vi "fgv_AOL_Globals Read.vi"(8 "error in (no error)":errorcluster) -> (0 "error out":errorcluster, 2 "AOL_Globals":T1={"Imaging Protocol"=enum."AOL Z-Stack", "Number of POI"=0, "Number of Miniscans"=0, "Number of Trials"=0, "Number of Cycles "=0, "# Averaged Frames"=0, "Laser power (%)"=0, "Pockels (V)"=0.0, "Acquisition Length (sec)"=0.0, "Fill time (us)"=0.0, "POI Dwell time (us)"=0.0, "Miniscan Dwell time per pixel (us)"=0.0, "PMT 1"=0.0, "PMT 2"=0.0, "Back Apperture (mA)"=0.0, "Frame Size"=512, "Center Frequency"=0.0, "Field of View (um)"=175.0, "Field of View (norm)"=175.0, "DwellTime (us)"=0.0, "Ref Dwell Time (us)"=0.0, "Wavelength (nm)"=0.0, "Zoom"=1.0, "AOL Z"=0.0, "AOL Mode"=enum."Raster", "GridXY"=0.0, "GridZ"=0.0, "TriggerPeriod (sec)"=0.0, "Number of Pixels in Miniscan"=0, "Experiment folder path"=path "", "X centre"=0.0, "Y centre"=0.0, "Angle (degrees)"=0.0, "Angle Xs (degrees)"=0.0, "Angle Ys (degrees)"=0.0, "Plane Mode"=0, "Threshold"=[], "Regenerate Chirps"=FALSE, "Rectangle ROI length (pixels)"=0, "Rectangle ROI height (pixels)"=0, "AOD fill"=4900, "StartupDelay"=0, "Samples Wait after Trigger"=5080, "Slip Cycle"=600000, "Add Cycle"=TRUE, "Functional Mode"=enum."Point", "Z Start"=0.0, "Z Stop"=0.0, "# Planes"=0, "Total Pixels"=0, "Variable Miniscan Pixels"=[], "Use Variable Length"=FALSE, "Use Variable Resolution"=FALSE, "Laser power (%) at Z Start"=0, "Laser power (%) at Z Stop"=0, "Ref Z Step"=0} {"Angle Ys (degrees)" format="%#.6g"; "Angle Xs (degrees)" format="%#.6g"; "Plane Mode" items=["XY Plane", "XZ Plane", "YZ Plane", "arbitraryplane"]; "Frame Size" items=["100X100"=100, "128X128"=128, "200X200"=200, "256X256"=256, "512X512"=512, "1024x1024"=1024, "2048x2048"=2048]; "Back Apperture (mA)" format="%#.6g"; "Pockels (V)" format="%#.6g"; "PMT 2" format="%#.6g"; "PMT 1" format="%#.6g"; "Angle (degrees)" format="%#.6g"; "POI Dwell time (us)" format="%#.6g"}, 3 "Imaging Protocol":T2)   [LabVIEW 2020]
uses:
  Typedefs/Controls/AOL_Globals.ctl
  Typedefs/Imaging Protocols enum.ctl
  Typedefs/Frame Size.ctl
  Typedefs/AOL modes.ctl
  Typedefs/Plane Mode.ctl
  Typedefs/Functional Mode.ctl
panel:
  # "<---- NOTE!  I don't think the PMT1\n          and PMT2 values are used. Elliminate."
  # "<---- NOTE!  Normalised FOV value"
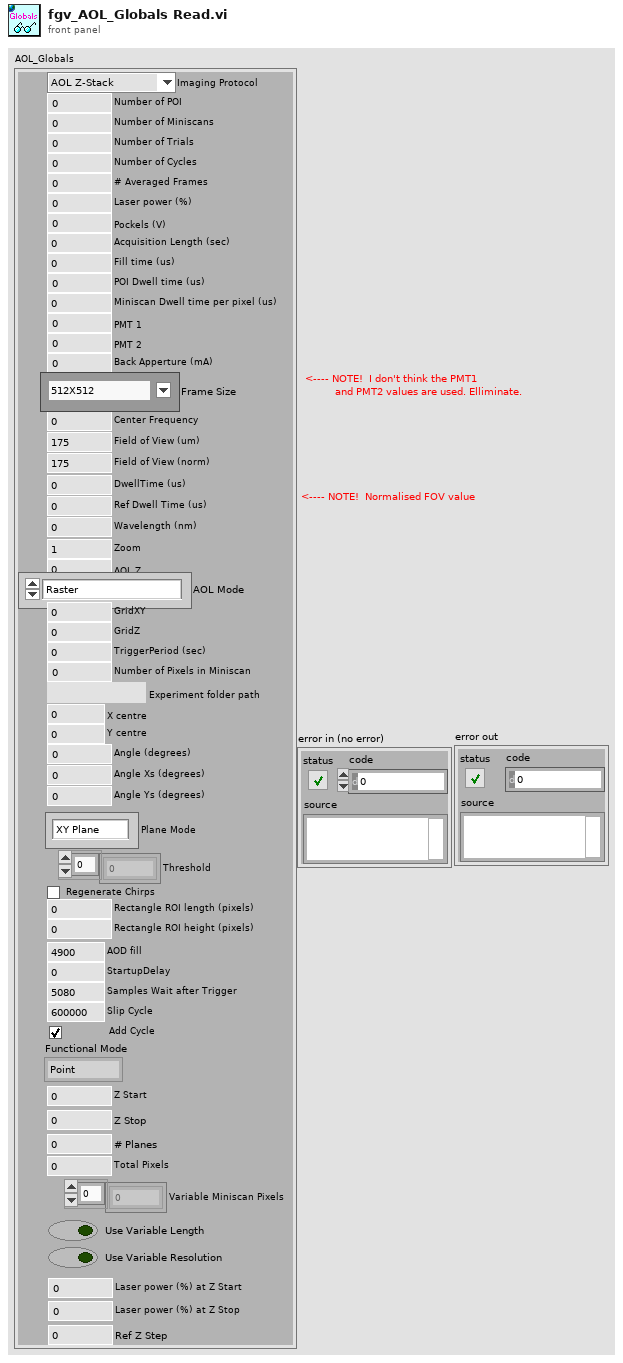
[diagram p1: front panel]
types:
  T1 = typedef "AOL_Globals.ctl" = cluster{"Imaging Protocol":T2, "Number of POI":u16, "Number of Miniscans":u16, "Number of Trials":u16, "Number of Cycles ":u64, "# Averaged Frames":u16, "Laser power (%)":u8, "Pockels (V)":dbl, "Acquisition Length (sec)":dbl, "Fill time (us)":dbl, "POI Dwell time (us)":dbl, "Miniscan Dwell time per pixel (us)":dbl, "PMT 1":dbl, "PMT 2":dbl, "Back Apperture (mA)":dbl, "Frame Size":T3, "Center Frequency":dbl, "Field of View (um)":dbl, "Field of View (norm)":dbl, "DwellTime (us)":dbl, "Ref Dwell Time (us)":dbl, "Wavelength (nm)":dbl, "Zoom":dbl, "AOL Z":dbl, "AOL Mode":T4, "GridXY":dbl, "GridZ":dbl, "TriggerPeriod (sec)":dbl, "Number of Pixels in Miniscan":u16, "Experiment folder path":path, "X centre":dbl, "Y centre":dbl, "Angle (degrees)":dbl, "Angle Xs (degrees)":dbl, "Angle Ys (degrees)":dbl, "Plane Mode":T5, "Threshold":u16[], "Regenerate Chirps":bool, "Rectangle ROI length (pixels)":u16, "Rectangle ROI height (pixels)":u16, "AOD fill":u16, "StartupDelay":i32, "Samples Wait after Trigger":u16, "Slip Cycle":u32, "Add Cycle":bool, "Functional Mode":T6, "Z Start":dbl, "Z Stop":dbl, "# Planes":i32, "Total Pixels":i32, "Variable Miniscan Pixels":u16[], "Use Variable Length":bool, "Use Variable Resolution":bool, "Laser power (%) at Z Start":u8, "Laser power (%) at Z Stop":u8, "Ref Z Step":i8}
  T2 = typedef "Imaging Protocols enum.ctl" = enum16{"AOL Z-Stack", "Motor Z Stack", "Parameter Sweep", "Functional Acquisition", "Single Plane Acquisition", "Volume Acquisition", "Live Imaging", "Live Plane Imaging", "Live Volume Imaging"}
  T3 = typedef "Frame Size.ctl" = u16
  T4 = typedef "AOL modes.ctl" = enum16{"Raster", "Structural", "Pointing", "Mini Scan", "Alignment"}
  T5 = typedef "Plane Mode.ctl" = u16
  T6 = typedef "Functional Mode.ctl" = enum16{"Point", "Line", "Patch", "Plane", "Volume"}
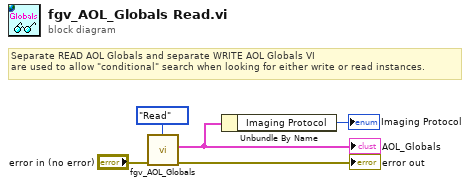
[diagram p0: block diagram]
diagram:
  # "Separate READ AOL Globals and separate WRITE AOL Globals VI \nare used to allow \"conditional\" search when looking for either write or read instances."
  n1 = call "fgv_AOL_Globals.vi"("error in (no error)"="error in (no error)", "Function"=enum16{"Intialize", "Write", "Read", "Clear"}."Read") -> ("error out"=→"error out":errorcluster, "AOL_Globals"=w1:T1)  [unwired: 8 in]
  "AOL_Globals" <- w1
  n2 = Unbundle By Name(w1) -> ("Imaging Protocol"=→"Imaging Protocol":T2)
